vi "WLAN - TV - RW - UTIL - ClusterToArray.vi"(7 "TV Paramaters":T1) -> (8 "TV_Parameters(1-D array)":string[](array[string]))   [LabVIEW 2012]
uses:
  Includes/WLAN - TV - RW - INC - TV_Parameters.ctl
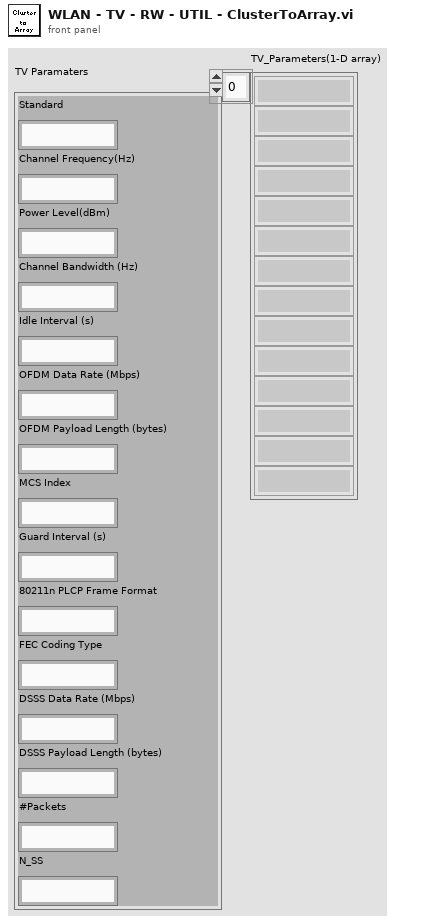
[diagram p1: front panel]
types:
  T1 = typedef "WLAN - TV - RW - INC - TV_Parameters.ctl" = cluster{"Standard ":string, "Channel Frequency(Hz)":string, "Power Level(dBm)":string, "Channel Bandwidth (Hz)":string, "Idle Interval (s)":string, "OFDM Data Rate (Mbps)":string, "OFDM Payload Length (bytes)":string, "MCS Index":string, "Guard Interval (s)":string, "80211n PLCP Frame Format":string, "FEC Coding Type":string, "DSSS Data Rate (Mbps)":string, "DSSS Payload Length (bytes)":string, "#Packets":string, "N_SS":string}
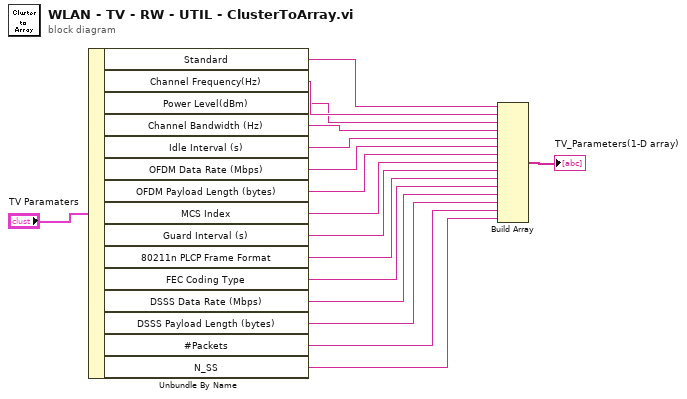
[diagram p0: block diagram]
diagram:
  n1 = Unbundle By Name("TV Paramaters") -> ("Standard"=w17:string, "Channel Frequency(Hz)"=w16:string, "Power Level(dBm)"=w15:string, "Channel Bandwidth (Hz)"=w14:string, "Idle Interval (s)"=w13:string, "OFDM Data Rate (Mbps)"=w12:string, "OFDM Payload Length (bytes)"=w11:string, "MCS Index"=w10:string, "Guard Interval (s)"=w9:string, "80211n PLCP Frame Format"=w8:string, "FEC Coding Type"=w7:string, "DSSS Data Rate (Mbps)"=w6:string, "DSSS Payload Length (bytes)"=w5:string, "#Packets"=w2:string, "N_SS"=w1:string)
  n2 = Build Array(w17, w16, w15, w14, w13, w12, w11, w10, w9, w8, w7, w6, w5, w2, w1) -> (→"TV_Parameters(1-D array)":string[])
